vi "LWXPS_PositionerMotorOutputOffsetGet.vi"(0 "XPS Reference IN":refnum<k24>, 2 "Positioner Name":string, 5 "LabVIEW error IN":errorcluster) -> (10 "XPS Reference OUT":refnum<k24>, 11 "LabVIEW error OUT":errorcluster, 12 "Returned error code":i32, 13 "XPS Error String":string, 14 "Primary DAC 1":dbl, 15 "Primary DAC 2":dbl, 16 "Primary DAC Differential Gain":dbl, 17 "Secondary DAC 1":dbl, 18 "Secondary DAC 2":dbl, 19 "Secondary DAC Differential Gain":dbl)   [LabVIEW 2014]
uses:
  D:/XPSQ8_LabView_Library/Development/Source/Dll/Newport.XPS.CommandInterface.dll
  Dll/Newport.XPS.CommandInterface.dll
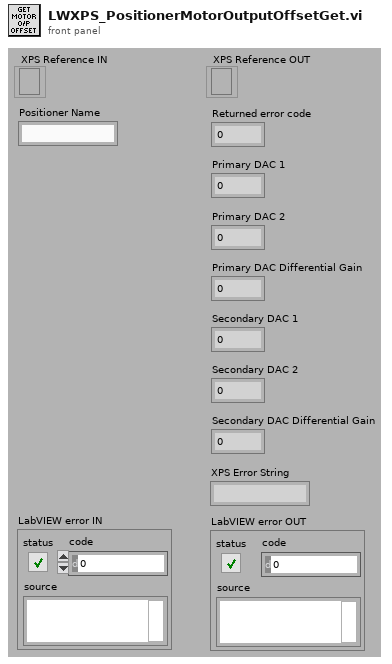
[diagram p1: front panel]
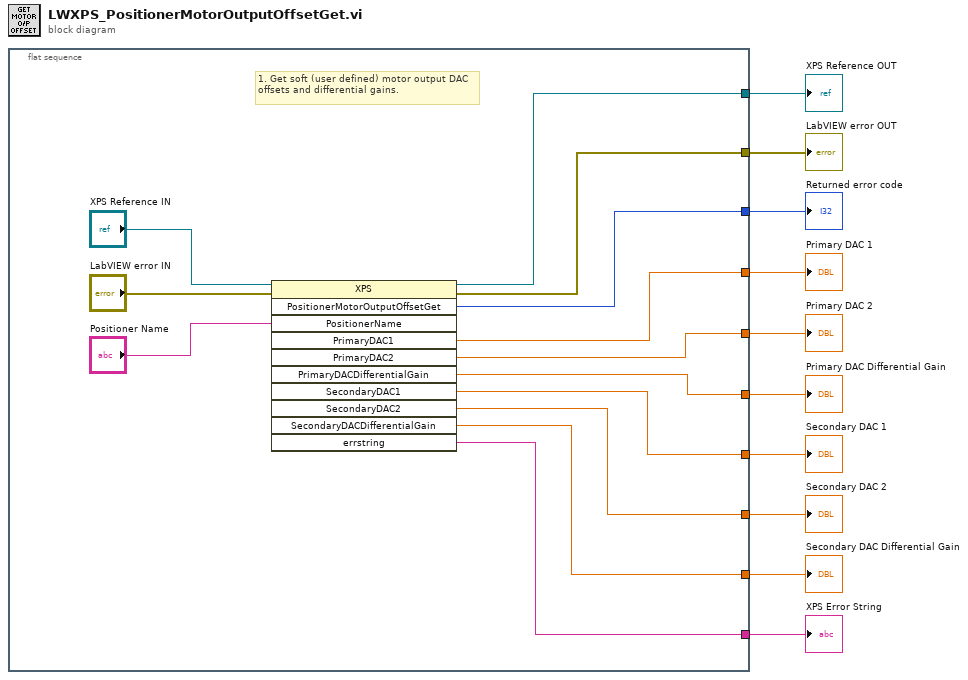
[diagram p0: block diagram]
diagram:
  n1 = flat-sequence {
    tunnel: [w21] -> w10
    tunnel: [w18] -> w9
    tunnel: [w22] -> w8
    tunnel: [w13] -> w1
    tunnel: [w16] -> w7
    tunnel: [w17] -> w4
    tunnel: [w15] -> w6
    tunnel: [w14] -> w5
    tunnel: [w12] -> w3
    tunnel: [w11] -> w2
    frame #0 {
      # "1. Get soft (user defined) motor output DAC offsets and differential gains."
      n2 = invoke class="XPS" method="PositionerMotorOutputOffsetGet"(reference="XPS Reference IN", error in="LabVIEW error IN", "PositionerName"="Positioner Name") -> (reference out=w21:refnum<k24>, error out=w18:errorcluster, "PositionerMotorOutputOffsetGet"=w22:i32, "PrimaryDAC1"=w13:dbl, "PrimaryDAC2"=w16:dbl, "PrimaryDACDifferentialGain"=w15:dbl, "SecondaryDAC1"=w14:dbl, "SecondaryDAC2"=w17:dbl, "SecondaryDACDifferentialGain"=w12:dbl, "errstring"=w11:string)  [unwired: 8 in, 1 out]
    }
  }
  "XPS Error String" <- w2
  "XPS Reference OUT" <- w10
  "LabVIEW error OUT" <- w9
  "Returned error code" <- w8
  "Primary DAC 2" <- w7
  "Primary DAC Differential Gain" <- w6
  "Secondary DAC 1" <- w5
  "Secondary DAC 2" <- w4
  "Secondary DAC Differential Gain" <- w3
  "Primary DAC 1" <- w1
